vi "bt_start_sub.vi"(0 "auto?":bool) -> (1 "connection ID":refnum<k31>, 2 "open error":errorcluster)   [LabVIEW 2012]
panel:
  out "address out":string
  out "service list":T1(array[cluster])
  out "device list":T2(array[cluster])
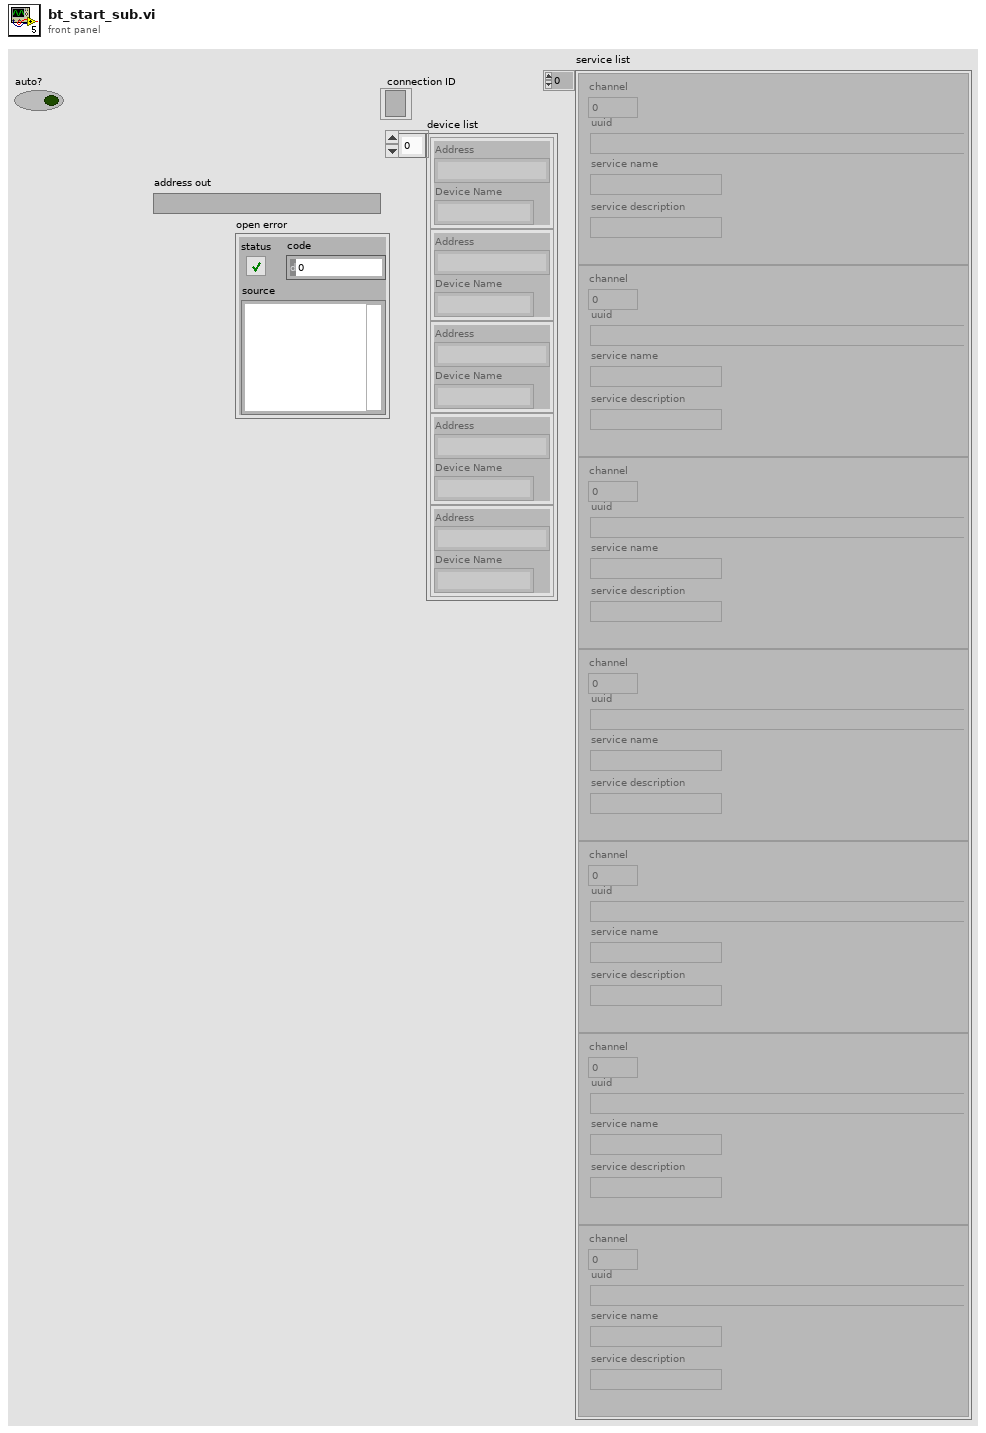
[diagram p1: front panel]
types:
  T1 = cluster{"channel":u16, "uuid":string, "service name":string, "service description":string}[]
  T2 = cluster{"Address":string, "Device Name":string}[]
  T3 = cluster{"channel":u16, "uuid":string, "service name":string, "service description":string}
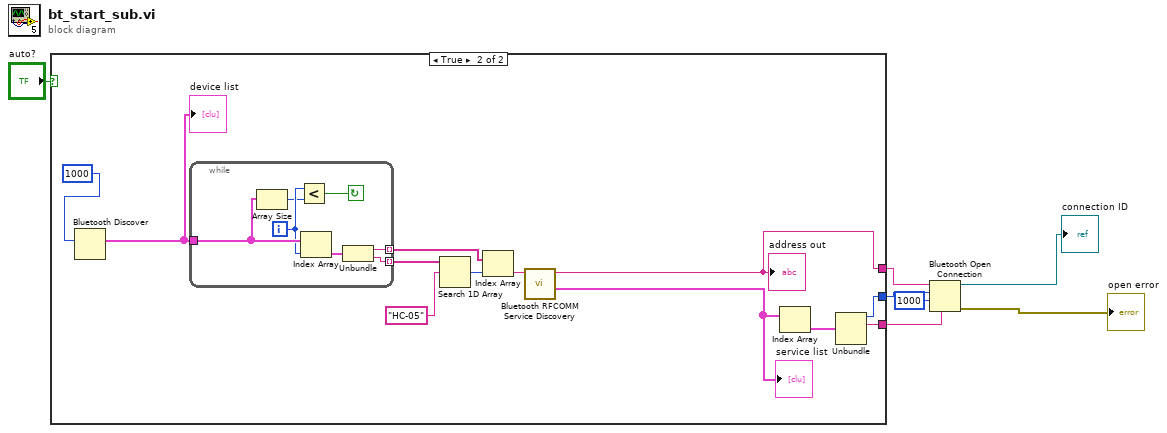
[diagram p0: block diagram]
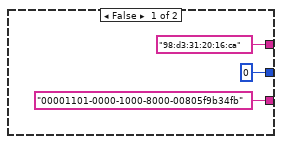
[diagram p2: hidden frame]
diagram:
  n1 = case shown="True" "auto?" {
    tunnel: ["00001101-0000-1000-8000-00805f9b34fb" ("uuid") w20] -> w2
    tunnel: [u16 0 ("channel") w19] -> w7
    tunnel: ["98:d3:31:20:16:ca" ("address out") w12] -> w6
    frame False {
    }
    frame True {
      n2 = Bluetooth Discover(10:1000 ("time limit ms (10000)")) -> (2:w18:T2)  [unwired: 1 in, 2 out]
      "device list" <- w18
      n3 = while {
        tunnel: w18 -> [w29]
        tunnel: [w24] -> w14 mode=indexing
        tunnel: [w23] -> w17 mode=indexing
        i -> [w28]
        stop <- w26 continue-if-true
        n4 = Array Size(array=w29) -> (size(s)=w27:i32)
        n5 = Less?(x=w28, y=w27) -> (x < y?=w26:bool)
        n6 = Index Array(array=w29, index=w28) -> (element=w25:cluster{"Address":string, "Device Name":string})
        n7 = Unbundle(w25) -> ("Address"=w24:string, "Device Name"=w23:string)
      }
      n8 = Search 1D Array(1D array=w17, element="HC-05") -> (index of element=w15:i32)  [unwired: 1 in]
      n9 = Index Array(array=w14, index=w15) -> (element=w13:string)
      n10 = call <vilib>:"Bluetooth RFCOMM Service Discovery.vi"("address in"=w13) -> ("service list"=w22:T1, "address out"=w12:string)  [unwired: 3 in, 2 out]
      "service list" <- w22
      "address out" <- w12
      n11 = Index Array(array=w22) -> (element=w21:T3)  [unwired: 1 in]
      n12 = Unbundle(w21) -> ("channel"=w19:u16, "uuid"=w20:string)  [unwired: 2 out]
    }
  }
  n13 = Bluetooth Open Connection(6:w2, 9:1000 ("timeout ms (60000)"), 10:w7, 11:w6) -> (0:→"open error":errorcluster, 3:→"connection ID":refnum<k31>)  [unwired: 1 in]
